vi "Start Drag.vi"(0 "FSM.Edge in":refnum<class "FSM.Edge.lvclass">, 7 "dragged nodes":string[](array[string]), 9 "Grid size":dbl) -> (4 "FSM.Edge out":refnum<class "FSM.Edge.lvclass">)   [LabVIEW 2020, in "FSM.Edge.lvclass"]
uses:
  FSM.Edge.lvclass
  FSM.Edge.lvclass/FSM.Edge.ctl
  FSM.Label/FSM.Label.lvclass/FSM.Label.ctl
  FSM.Label/Read Location.vi
  FSM.Label/FSM.Label.lvclass
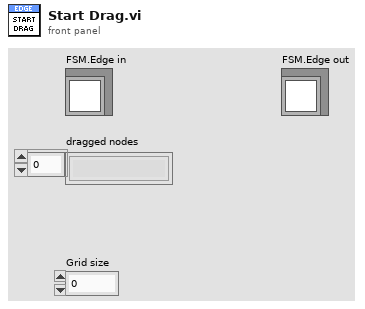
[diagram p1: front panel]
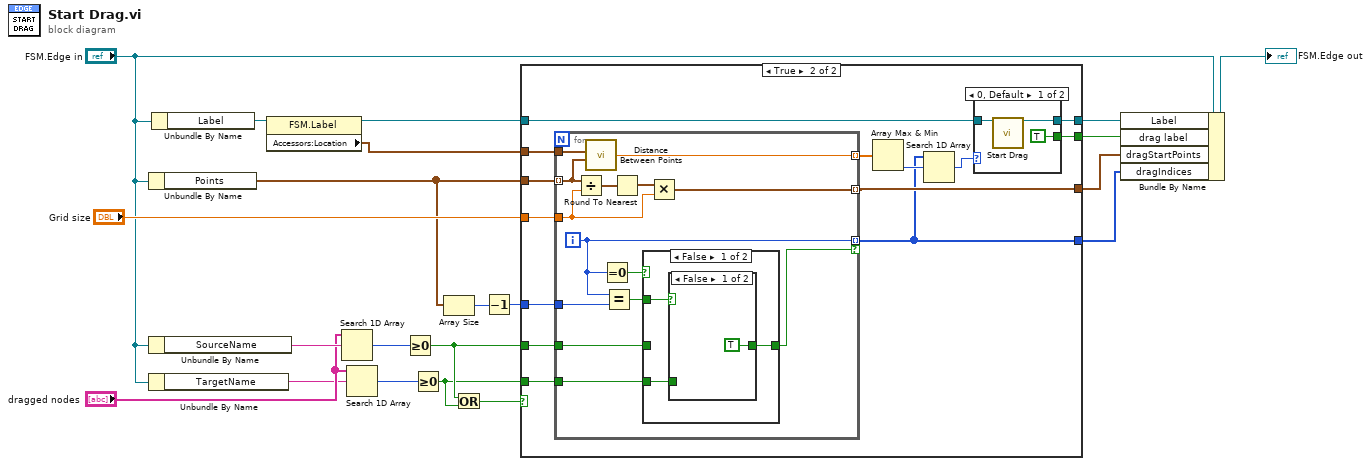
[diagram p0: block diagram]
diagram:
  n1 = Unbundle By Name("FSM.Edge in") -> ("Points"=w20:cluster{"x":i16, "y":i16}[])
  n2 = Unbundle By Name("FSM.Edge in") -> ("SourceName"=w5:string)
  n3 = Unbundle By Name("FSM.Edge in") -> ("TargetName"=w2:string)
  n4 = Unbundle By Name("FSM.Edge in") -> ("Label"=w17:refnum<class "FSM.Label.lvclass">)
  n5 = property class="FSM.Label"(reference=w17) -> (reference out=w15:refnum<class "FSM.Label.lvclass">, "Accessors:Location"=w16:cluster{"x":i16, "y":i16})  [unwired: 1 in, 1 out]
  n6 = Search 1D Array(1D array="dragged nodes", element=w5) -> (index of element=w4:i32)  [unwired: 1 in]
  n7 = Search 1D Array(1D array="dragged nodes", element=w2) -> (index of element=w1:i32)  [unwired: 1 in]
  n8 = Greater Or Equal To 0?(x=w4) -> (x >= 0?=w10:bool)
  n9 = Greater Or Equal To 0?(x=w1) -> (x >= 0?=w9:bool)
  n10 = Array Size(array=w20) -> (size(s)=w11:i32)
  n11 = Or(x=w10, y=w9) -> (x .or. y?=w12:bool)
  n12 = Decrement(x=w11) -> (x-1=w6:i32)
  n13 = case shown="True" w12 {
    tunnel: "Grid size" -> [_ w36]
    tunnel: w20 -> [_ w35]
    tunnel: [_ w34] -> w14
    tunnel: [_ w27] -> w13
    tunnel: w6 -> [_ w33]
    tunnel: w10 -> [_ w32]
    tunnel: w9 -> [_ w31]
    tunnel: w16 -> [_ w30]
    tunnel: w15 -> [w22 w26]
    tunnel: [w22 w24] -> w8
    tunnel: [_ w23] -> w7
    frame False {
    }
    frame True {
      n14 = for {
        tunnel: w36 -> [w54]
        tunnel: w35 -> [w45] mode=indexing
        tunnel: [w52] -> w34 mode=indexing
        tunnel: [w51] -> w27 mode=indexing if=w47
        tunnel: w33 -> [w50]
        tunnel: w32 -> [w42]
        tunnel: w31 -> [w41]
        tunnel: w30 -> [w44]
        tunnel: [w43] -> w29 mode=indexing
        i -> [w51]
        n15 = Divide(x=w45, y=w54) -> (x/y=w46:cluster{"x":dbl, "y":dbl})
        n16 = call "Distance Between Points.vi"("B"=w45, "A"=w44) -> ("distance"=w43:dbl)  [unwired: 4 in]
        n17 = Equal To 0?(x=w51) -> (x = 0?=w49:bool)
        n18 = Equal?(x=w51, y=w50) -> (x = y?=w48:bool)
        n19 = Round To Nearest(number=w46) -> (nearest integer value=w53:cluster{"x":dbl, "y":dbl})
        n20 = case shown="False" w49 {
          tunnel: w42 -> [_ w60]
          tunnel: [w55 w60] -> w47
          tunnel: w48 -> [w57 _]
          tunnel: w41 -> [w56 _]
          frame False {
            n21 = case shown="False" w57 {
              tunnel: w56 -> [_ w59]
              tunnel: [TRUE w59] -> w55
              frame False {
              }
              frame True {
              }
            }
          }
          frame True {
          }
        }
        n22 = Multiply(x=w53, y=w54) -> (x*y=w52:cluster{"x":dbl, "y":dbl})
      }
      n23 = Array Max & Min(array=w29) -> (min index (indices)=w28:i32)  [unwired: 3 out]
      n24 = Search 1D Array(1D array=w27, element=w28) -> (index of element=w25:i32)  [unwired: 1 in]
      n25 = case shown="0, Default" w25 {
        tunnel: w26 -> [w39 w40]
        tunnel: [w38 w40] -> w24
        tunnel: [TRUE _] -> w23
        frame 0, Default {
          n26 = call "Start Drag.vi"("FSM.Label In"=w39) -> ("FSM.Label Out"=w38:refnum<class "FSM.Label.lvclass">)  [unwired: 14 in]
        }
        frame -1 {
        }
      }
    }
  }
  n27 = Bundle By Name(cluster="FSM.Edge in", "Label"=w8, "drag label"=w7, "dragStartPoints"=w14, "dragIndices"=w13) -> (→"FSM.Edge out":refnum<class "FSM.Edge.lvclass">)
